vi "fpga_LineInputs-Conn3-Set3.vi"() -> (0 "DataLines":T1)   [LabVIEW 2011]
uses:
  <vilib>/rvi/eio/common/nirviEmuTemplateMethod_errors.vi
  <vilib>/eio/EIONode/EIONode.xnode
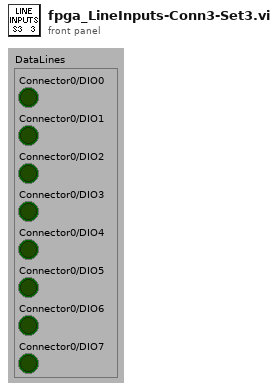
[diagram p1: front panel]
types:
  T1 = cluster{"Connector0/DIO0":bool, "Connector0/DIO1":bool, "Connector0/DIO2":bool, "Connector0/DIO3":bool, "Connector0/DIO4":bool, "Connector0/DIO5":bool, "Connector0/DIO6":bool, "Connector0/DIO7":bool}
  T2 = cluster{"Connector3/DIO24":bool, "Connector3/DIO25":bool, "Connector3/DIO26":bool, "Connector3/DIO27":bool, "Connector3/DIO28":bool, "Connector3/DIO29":bool, "Connector3/DIO30":bool, "Connector3/DIO31":bool}
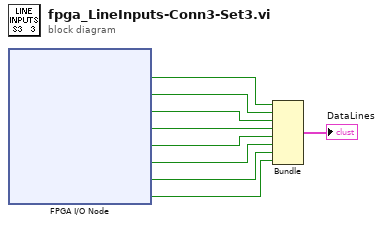
[diagram p0: block diagram]
diagram:
  n1 = xnode "FPGA I/O Node"() -> ("Connector3/DIO24"=w9:bool, "Connector3/DIO25"=w8:bool, "Connector3/DIO26"=w7:bool, "Connector3/DIO27"=w6:bool, "Connector3/DIO28"=w5:bool, "Connector3/DIO29"=w4:bool, "Connector3/DIO30"=w3:bool, "Connector3/DIO31"=w2:bool)  [unwired: 8 in, 8 out]
  n2 = Bundle("Connector3/DIO24"=w9, "Connector3/DIO25"=w8, "Connector3/DIO26"=w7, "Connector3/DIO27"=w6, "Connector3/DIO28"=w5, "Connector3/DIO29"=w4, "Connector3/DIO30"=w3, "Connector3/DIO31"=w2) -> (→"DataLines":T2)  [unwired: 1 in]
